vi "WriteAddress.vi"(0 "Task in":refnum<class "WaveformTask.lvclass">, 5 "address":u64, 7 "data":u64, 11 "error in (no error)":errorcluster, 12 "timeout (5000 ms)":i32=5000) -> (4 "Task out":refnum<class "WaveformTask.lvclass">, 15 "error out":errorcluster)   [LabVIEW 2017, in "WaveformTask.lvclass"]
uses:
  WaveformTask.lvclass
  WaveformTask.lvclass/WaveformTask.ctl
  <instrlib>/_niInstr/FIFO Register Bus/v1/Host/niInstr FIFO Register Bus v1 Host.lvclass
  C:/Program Files (x86)/National Instruments/LabVIEW 2017/instr.lib/_niInstr/Instruction Framework/v1/Host/Instruction Target/niInstr Instruction Target v1 Host.lvclass
  <instrlib>/_niInstr/Instruction Framework/v1/Host/Instruction Target/niInstr Instruction Target v1 Host.lvclass
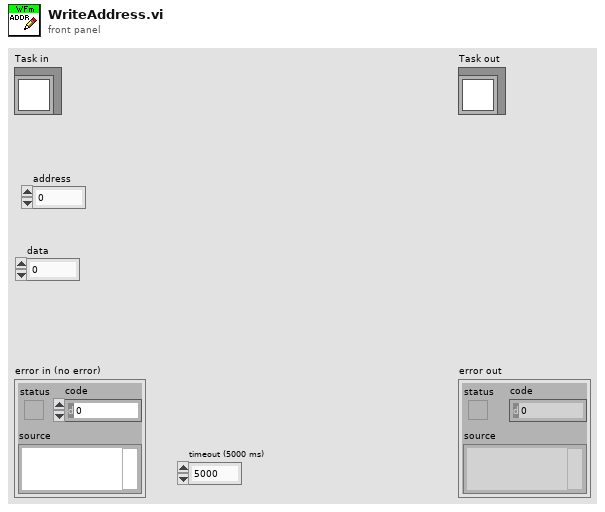
[diagram p1: front panel]
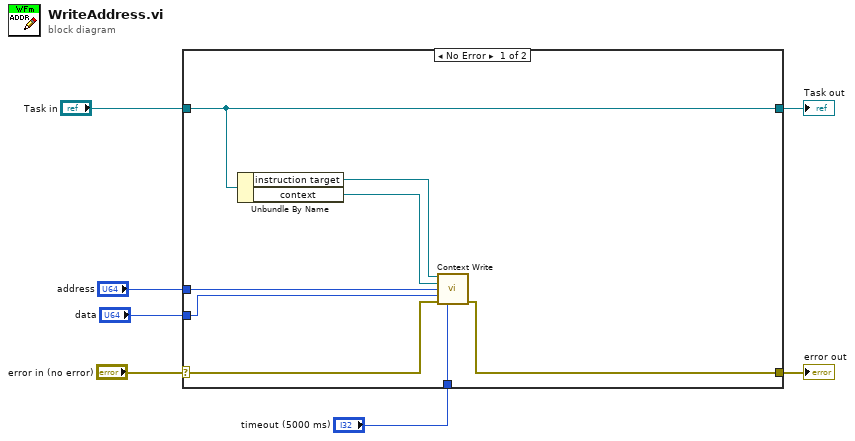
[diagram p0: block diagram]
diagram:
  n1 = case shown="No Error" "error in (no error)" {
    selector: "error in (no error)" -> [w13 w17]
    tunnel: [w12 w17] -> w6
    tunnel: [w9 w16] -> w4
    tunnel: "Task in" -> [w9 w16]
    tunnel: "address" -> [w11 _]
    tunnel: "data" -> [w10 _]
    tunnel: "timeout (5000 ms)" -> [w8 _]
    frame No Error {
      n2 = Unbundle By Name(w9) -> ("instruction target"=w15:refnum<class "niInstr FIFO Register Bus v1 Host.lvclass">, "context"=w14:refnum<class "niInstr Instruction Framework Context v1 Host.lvclass">)
      n3 = call <instrlib>:"Context Write.vi"("instruction target in"=w15, "context in"=w14, "address"=w11, "data"=w10, "error in"=w13, "timeout (5000 ms)"=w8) -> ("error out"=w12:errorcluster)  [unwired: 7 in, 2 out]
    }
    frame Error {
    }
  }
  "error out" <- w6
  "Task out" <- w4
